vi "Multiplier 1.vi"(8 "Lower Slope":dbl, 10 "Input":dbl, 11 "Threshold":dbl) -> (2 "Output":dbl)   [LabVIEW 2012]
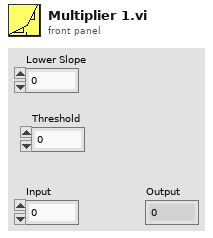
[diagram p1: front panel]
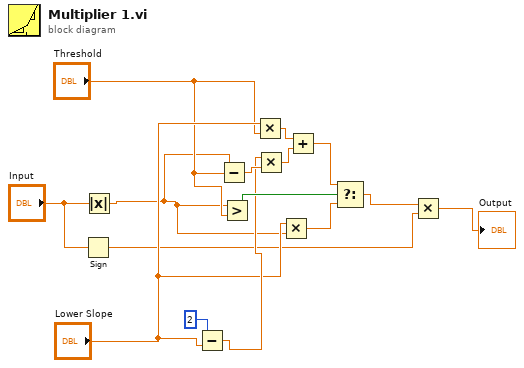
[diagram p0: block diagram]
diagram:
  n1 = Sign(1:"Input") -> (0:w3:dbl)
  n2 = Absolute Value(x="Input") -> (abs(x)=w1:dbl)
  n3 = Subtract(x=2, y="Lower Slope") -> (x-y=w9:dbl)
  n4 = Subtract(x=w1, y="Threshold") -> (x-y=w13:dbl)
  n5 = Greater?(x=w1, y="Threshold") -> (0:w12:bool)
  n6 = Multiply(x="Lower Slope", y="Threshold") -> (x*y=w15:dbl)
  n7 = Multiply(x=w9, y=w13) -> (x*y=w14:dbl)
  n8 = Multiply(x="Lower Slope", y=w1) -> (x*y=w10:dbl)
  n9 = Add(x=w15, y=w14) -> (x+y=w11:dbl)
  n10 = Select(t=w11, s=w12, f=w10) -> (s? t:f=w5:dbl)
  n11 = Multiply(x=w5, y=w3) -> (x*y=→"Output":dbl)
